vi "UV-VIS SetBaselineClamp.vi"(3 "error in (no error)":errorcluster, 4 "state":bool, 5 "Control in":refnum<class "UV-VIS.lvclass">) -> (0 "error out":errorcluster, 1 "DLL error code":u32, 2 "Control out":refnum<class "UV-VIS.lvclass">)   [LabVIEW 2015, in "UV-VIS.lvclass"]
doc: "This function turns on and off the baseline clamp functionality within the SDK. With this feature enabled the baseline level of each scan in a kinetic series will be more consistent across the sequence.\n\n<B>Parameter:</B>\nstate - Enables/Disables Baseline clamp functionality\n Valid values:\n FALSE – Disable Baseline Clamp\n TRUE – Enable Baseline Clamp\n\n<B>Error codes:</B>\nDRV_SUCCESS - Parameters set.\nDRV_NOT_INITIALIZED - System not initialized.\nDRV_ACQUIRING - Acquisition in progress.\nDRV_P1INVALID - State parameter was not zero or one."
uses:
  UV-VIS.lvclass
  Detector.lvclass/Detector.ctl
  Detector.lvclass
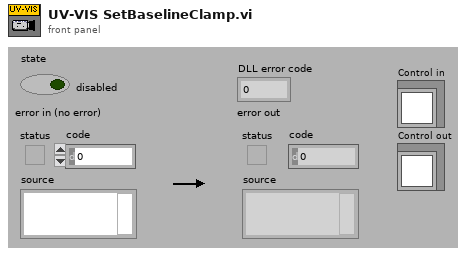
[diagram p1: front panel]
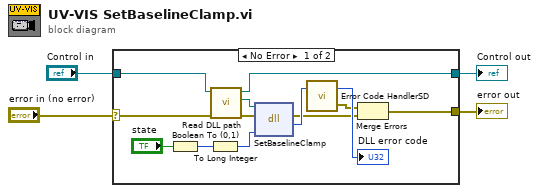
[diagram p0: block diagram]
diagram:
  n1 = case shown="No Error" "error in (no error)" {
    selector: "error in (no error)" -> [w12 w19]
    tunnel: [w6 w19] -> w3
    tunnel: [w5 w18] -> w2
    tunnel: "Control in" -> [w11 w18]
    frame No Error {
      n2 = Boolean To (0,1)(Boolean="state") -> (0, 1=w14:i16)
      n3 = To Long Integer(number=w14) -> (32bit integer=w13:i32)
      n4 = call "Read DLL path.vi"("error in (no error)"=w12, "Detector in"=w11) -> ("error out"=w10:errorcluster, "DLL path"=w9:path, "Detector out"=w5:refnum<class "UV-VIS.lvclass">)  [unwired: 7 in]
      n5 = dll-call lib="S:/TRANCON/DLL/atmcd32d.dll" fn="SetBaselineClamp"(path in=w9, error in=w10, "state"=w13) -> (error out=w8:errorcluster, "return type"=w17:u32)  [unwired: 2 in, 1 out]
      n6 = call "Error Code HandlerSD.vi"("DLL error code"=w17) -> ("error out"=w7:errorcluster, "dup DLL error code"=→"DLL error code":u32)  [unwired: 1 out]
      n7 = Merge Errors(w7, w8) -> (w6:errorcluster)
    }
    frame Error {
    }
  }
  "error out" <- w3
  "Control out" <- w2
